vi "Pressure_Multiplexer.vi"() -> (0 "DAQ Error":errorcluster)   [LabVIEW 2015]
uses:
  Pressure_Multiplexer/Software/EnFlo specific/Ctls/Cmd list.ctl
  Globals/Meas_global.vi
  Pressure_Multiplexer/Software/EnFlo specific/Globals/PressureMultiplexer global.vi
  PWA/PWAtasksGLOBAL.vi
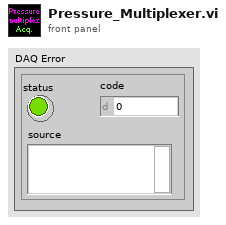
[diagram p1: front panel]
types:
  T1 = typedef "Ch_and_Spans.ctl" = cluster{"high limit (10V)":sgl, "low limit (-10V)":sgl, "Ch No":i16, "Var name":string, "Use Latest Calib":bool}
  T2 = typedef "Cmd list.ctl" = string
  T3 = typedef "Data values, Mode 0 (for datalog).ctl" = cluster{"Time Stamp":timestamp, "dt (us)":sgl, "dt_warn":u8, "Pressures":sgl[], "Statuses":u8[]}
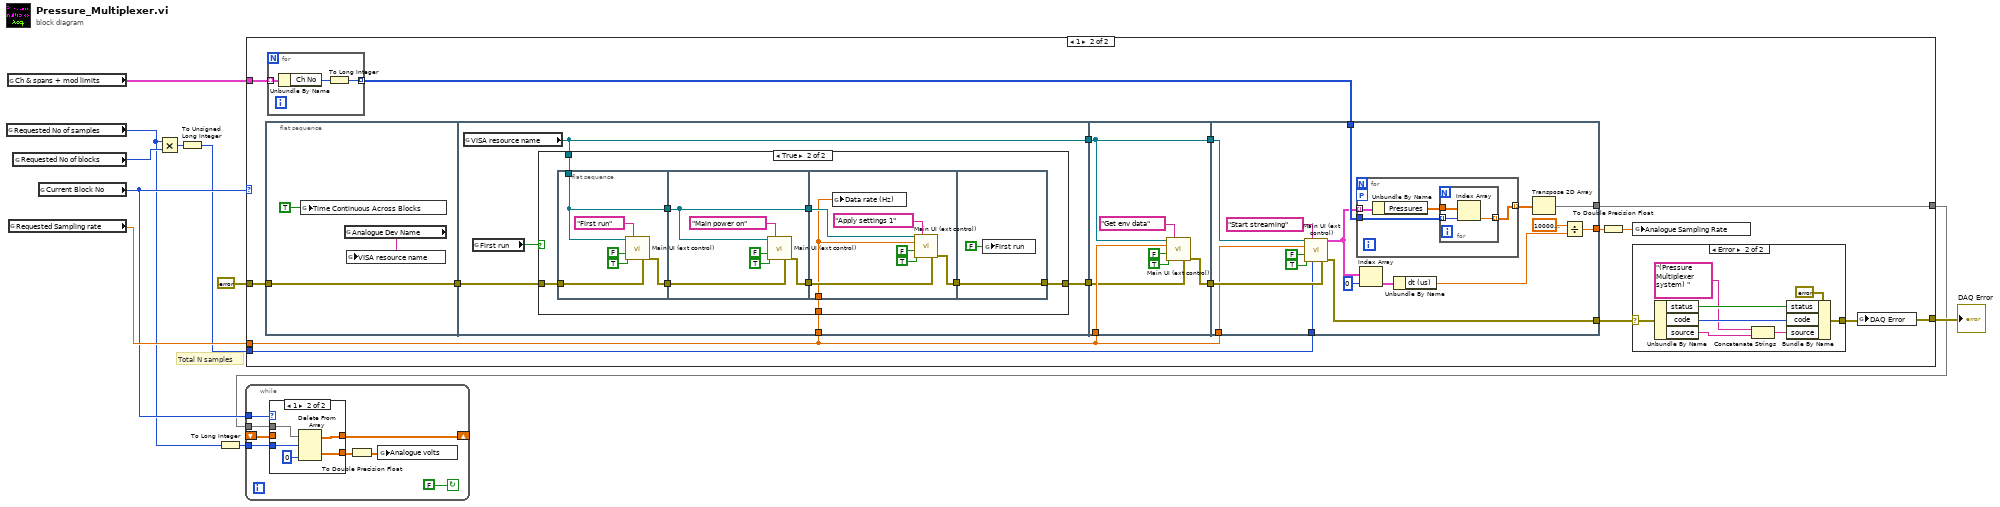
[diagram p0: block diagram]
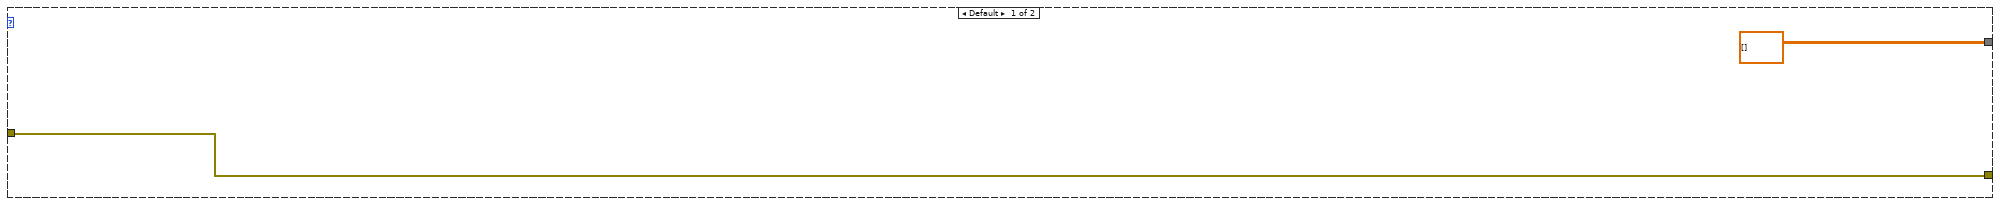
[diagram p2: hidden frame]
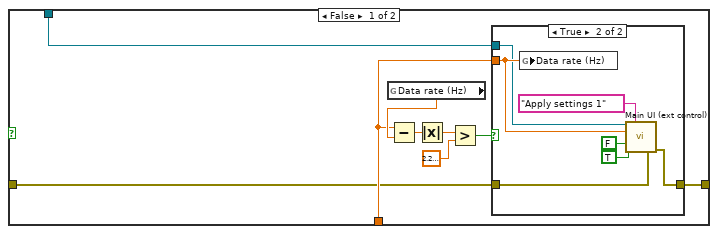
[diagram p3: hidden frame]
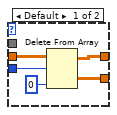
[diagram p6: hidden frame]
diagram:
  # "Total N samples"
  n1 = global read "Meas_global.vi" "Requested No of samples"() -> (w3:i32)
  n2 = global read "Meas_global.vi" "Ch & spans + mod limits"() -> (w9:T1[])
  n3 = global read "Meas_global.vi" "Requested Sampling rate"() -> (w11:dbl)
  n4 = global read "Meas_global.vi" "Requested No of blocks"() -> (w7:i32)
  n5 = global read "Meas_global.vi" "Current Block No"() -> (w6:i32)
  n6 = Multiply(x=w3, y=w7) -> (x*y=w8:i32)
  n7 = To Unsigned Long Integer(number=w8) -> (unsigned 32bit integer=w5:u32)
  n8 = To Long Integer(number=w3) -> (32bit integer=w4:i32)
  n9 = case shown="1" w6 {
    tunnel: w9 -> [_ w26]
    tunnel: [w13 w25] -> w10
    tunnel: errorcluster {"status"=FALSE, "code"=0, "source"=""} ("Error in") -> [w13 w22]
    tunnel: w5 -> [_ w21]
    tunnel: w11 -> [_ w16]
    tunnel: [sgl[][] [] w18] -> w2
    frame Default {
    }
    frame 1 {
      n10 = flat-sequence {
        tunnel: w22 -> [w31]
        tunnel: [w31] -> w17
        tunnel: [w34] -> w15
        tunnel: w17 -> [w35]
        tunnel: w16 -> [w33]
        tunnel: [w32] -> w14
        tunnel: w15 -> [w86]
        tunnel: [w87] -> w27
        tunnel: [w86] -> w28
        tunnel: w16 -> [w85]
        tunnel: w14 -> [w84]
        tunnel: w24 -> [w107]
        tunnel: [w93] -> w20
        tunnel: [w100] -> w18
        tunnel: [w106] -> w23
        tunnel: w28 -> [w96]
        tunnel: w27 -> [w95]
        tunnel: w21 -> [w92]
        tunnel: w16 -> [w91]
        frame #0 {
          n11 = global write "Meas_global.vi" "Time Continuous Across Blocks"(TRUE ("Time Continuous across Blocks")) -> ()
          n12 = global read "PWAtasksGLOBAL.vi" "Analogue Dev Name"() -> (w30:string)
          n13 = global write "PressureMultiplexer global.vi" "VISA resource name"(w30) -> ()
        }
        frame #1 {
          n14 = global read "PressureMultiplexer global.vi" "VISA resource name"() -> (w34:refnum<visa-resource-name>)
          n15 = global read "PressureMultiplexer global.vi" "First run"() -> (w36:bool)
          n16 = case shown="True" w36 {
            tunnel: w34 -> [w39 w62]
            tunnel: [w37 w61] -> w32
            tunnel: w35 -> [w38 w60]
            tunnel: w33 -> [w40 w54]
            frame False {
              n17 = global read "PressureMultiplexer global.vi" "Data rate (Hz)"() -> (w45:dbl)
              n18 = Subtract(x=w40, y=w45) -> (x-y=w42:dbl)
              n19 = Absolute Value(x=w42) -> (abs(x)=w43:dbl)
              n20 = Greater?(x=w43, y=2.220446049250313e-16) -> (0:w41:bool)
              n21 = case shown="True" w41 {
                tunnel: w38 -> [w46 w48]
                tunnel: [w46 w50] -> w37
                tunnel: w40 -> [_ w49]
                tunnel: w39 -> [_ w47]
                frame False {
                }
                frame True {
                  n22 = global write "PressureMultiplexer global.vi" "Data rate (Hz)"(w49) -> ()
                  n23 = call "Main UI (ext control).vi"("Serial port"=w47, "Command"=T2 "Apply settings 1", "Data rate (Hz)"=w49, "Wait for HW trigger"=FALSE, "Finite samples"=TRUE, "Error in"=w48) -> ("Error out"=w50:errorcluster)  [unwired: 8 in, 1 out]
                }
              }
            }
            frame True {
              n24 = flat-sequence {
                tunnel: w62 -> [w63]
                tunnel: w60 -> [w64]
                tunnel: [w65] -> w59
                tunnel: [w63] -> w58
                tunnel: w59 -> [w71]
                tunnel: w58 -> [w69]
                tunnel: [w70] -> w57
                tunnel: [w69] -> w55
                tunnel: w57 -> [w78]
                tunnel: [w77] -> w56
                tunnel: w55 -> [w76]
                tunnel: w54 -> [w75]
                tunnel: [w83] -> w61
                tunnel: w56 -> [w83]
                frame #0 {
                  n25 = call "Main UI (ext control).vi"("Serial port"=w63, "Command"=T2 "First run", "Wait for HW trigger"=FALSE, "Finite samples"=TRUE, "Error in"=w64) -> ("Error out"=w65:errorcluster)  [unwired: 9 in, 1 out]
                }
                frame #1 {
                  n26 = call "Main UI (ext control).vi"("Serial port"=w69, "Command"=T2 "Main power on", "Wait for HW trigger"=FALSE, "Finite samples"=TRUE, "Error in"=w71) -> ("Error out"=w70:errorcluster)  [unwired: 9 in, 1 out]
                }
                frame #2 {
                  n27 = global write "PressureMultiplexer global.vi" "Data rate (Hz)"(w75) -> ()
                  n28 = call "Main UI (ext control).vi"("Serial port"=w76, "Command"=T2 "Apply settings 1", "Data rate (Hz)"=w75, "Wait for HW trigger"=FALSE, "Finite samples"=TRUE, "Error in"=w78) -> ("Error out"=w77:errorcluster)  [unwired: 8 in, 1 out]
                }
                frame #3 {
                  n29 = global write "PressureMultiplexer global.vi" "First run"(FALSE ("First run")) -> ()
                }
              }
            }
          }
        }
        frame #2 {
          n30 = call "Main UI (ext control).vi"("Serial port"=w86, "Command"=T2 "Get env data", "Data rate (Hz)"=w85, "Wait for HW trigger"=FALSE, "Finite samples"=TRUE, "Error in"=w84) -> ("Error out"=w87:errorcluster)  [unwired: 8 in, 1 out]
        }
        frame #3 {
          n31 = call "Main UI (ext control).vi"("Serial port"=w96, "Command"=T2 "Start streaming", "Data rate (Hz)"=w91, "Wait for HW trigger"=FALSE, "Finite samples"=TRUE, "N samples"=w92, "Error in"=w95) -> ("P data (mode 0)"=w94:T3[], "Error out"=w93:errorcluster)  [unwired: 7 in]
          n32 = for {
            tunnel: [w108] -> w104 mode=indexing
            tunnel: w94 -> [w111] mode=indexing
            tunnel: w107 -> [w110]
            workers-P: _ -> [_]
            n33 = Unbundle By Name(w111) -> ("Pressures"=w109:sgl[])
            n34 = for {
              tunnel: w110 -> [w114] mode=indexing
              tunnel: w109 -> [w113]
              tunnel: [w112] -> w108 mode=indexing
              n35 = Index Array(array=w113, index=w114) -> (element=w112:sgl)
            }
          }
          n36 = Index Array(array=w94, index=0) -> (element=w102:T3)
          n37 = Unbundle By Name(w102) -> ("dt (us)"=w101:sgl)
          n38 = Transpose 2D Array(2D array=w104) -> (transposed array=w100:sgl[][])
          n39 = Divide(x=sgl 1000000.0 ("y"), y=w101) -> (x/y=w106:sgl)
        }
      }
      n40 = for {
        tunnel: w26 -> [w117] mode=indexing
        tunnel: [w115] -> w24 mode=indexing
        n41 = Unbundle By Name(w117) -> ("Ch No"=w116:i16)
        n42 = To Long Integer(number=w116) -> (32bit integer=w115:i32)
      }
      n43 = To Double Precision Float(number=w23) -> (double precision float=w19:dbl)
      n44 = global write "Meas_global.vi" "Analogue Sampling Rate"(w19) -> ()
      n45 = case shown="Error" w20 {
        selector: w20 -> [w118 w119]
        tunnel: [w118 w126] -> w25
        frame No Error {
        }
        frame Error {
          n46 = Unbundle By Name(w119) -> ("status"=w124:bool, "code"=w123:i32, "source"=w122:string)
          n47 = Concatenate Strings("(Pressure Multiplexer system) " ("source"), w122) -> (w120:string)
          n48 = Bundle By Name(cluster=errorcluster {"status"=FALSE, "code"=0, "source"=""} ("DAQ Error"), "status"=w124, "code"=w123, "source"=w120) -> (w126:errorcluster)
        }
      }
      n49 = global write "Meas_global.vi" "DAQ Error"(w25) -> ()
    }
  }
  "DAQ Error" <- w10
  n50 = while {
    shift-right: [w131] -> _
    shift-left: _ -> [w134]
    tunnel: w6 -> [w133]
    tunnel: w4 -> [w132]
    tunnel: w2 -> [w130]
    stop <- FALSE continue-if-true
    n51 = case shown="1" w133 {
      tunnel: w134 -> [w138 _]
      tunnel: w132 -> [w137 w143]
      tunnel: [w136 w142] -> w131
      tunnel: w130 -> [_ w141]
      tunnel: [w135 w140] -> w128
      frame Default {
        n52 = Delete From Array(array=w138, length=w137, index (col)=0 ("disabled index (col)")) -> (deleted portion=w135:sgl[][], array with subset deleted=w136:sgl[][])  [unwired: 1 in]
      }
      frame 1 {
        n53 = Delete From Array(array=w141, length=w143, index (col)=0 ("disabled index (col)")) -> (deleted portion=w140:sgl[][], array with subset deleted=w142:sgl[][])  [unwired: 1 in]
      }
    }
    n54 = To Double Precision Float(number=w128) -> (double precision float=w127:dbl[][])
    n55 = global write "Meas_global.vi" "Analogue volts"(w127) -> ()
  }
